vi "DataPathGlobalVariable.vi"() -> ()   [LabVIEW 2013, in "main.lvlib"]
uses:
  main.lvlib
panel:
  in  "Current Measurement ID":string
  in  "DataPatientPath":path
  in  "DataPatientDatePath":path
  in  "Template Path":path
  in  "Graph Path":path
  in  "DatabasePath":string
  out "ReportPath":path
  out "DataPath":path
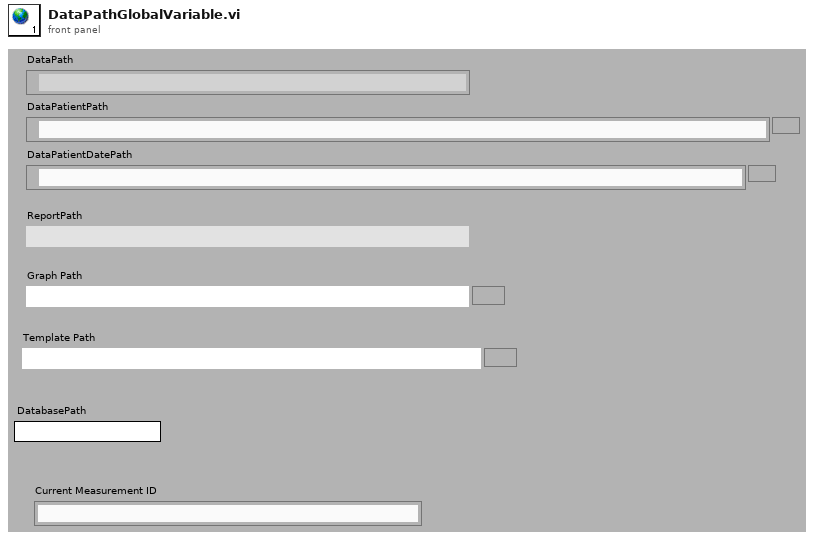
[diagram p1: front panel]
diagram:
